vi "Mode 2 Num.vi"(0 "Mode":cluster{"Run":bool, "Hold":bool, "Off":bool}) -> (1 "Mode":enum16{"Run", "Hold", "Off"}(ring), 2 "Mode Out":cluster{"Run":bool, "Hold":bool, "Off":bool})   [LabVIEW 2012]
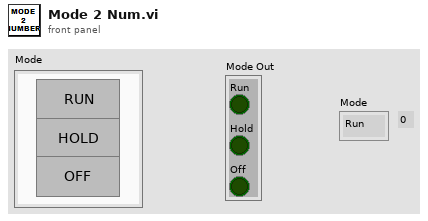
[diagram p1: front panel]
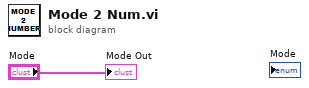
[diagram p0: block diagram]
diagram:
  "Mode Out" <- "Mode"
